vi "LVJSON Load.vi"(8 "error in (no error)":errorcluster, 11 "JSON in":string) -> (0 "error out":errorcluster, 1 "Empty?":bool, 3 "Root Element out":T1)   [LabVIEW 2018, in "labview_json.lvlib"]
uses:
  labview_json.lvlib
  Element Type.ctl
  Element.ctl
  <vilib>/regexp/Match Regular Expression.xnode
  <vilib>/ErrorRing/Error Ring.xnode
  <vilib>/Utility/error.llb/Error Cluster From Error Code.vi
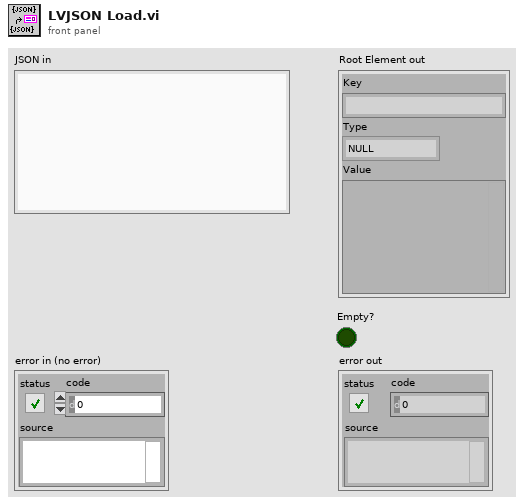
[diagram p1: front panel]
types:
  T1 = typedef "labview_json.lvlib/Element.ctl" = cluster{"Key":string, "Type":T2, "Value":variant}
  T2 = typedef "labview_json.lvlib/Element Type.ctl" = enum8{"NULL", "BOOL", "INT", "UINT", "FLOAT", "STRING", "ARRAY", "OBJECT", "SKIP"}
  T3 = cluster{"Kind":enum8{"Root", "Object", "Array"}, "Name":string, "Values":T1[]}[]
  T4 = cluster{"Kind":enum8{"Root", "Object", "Array"}, "Name":string, "Values":T1[]}
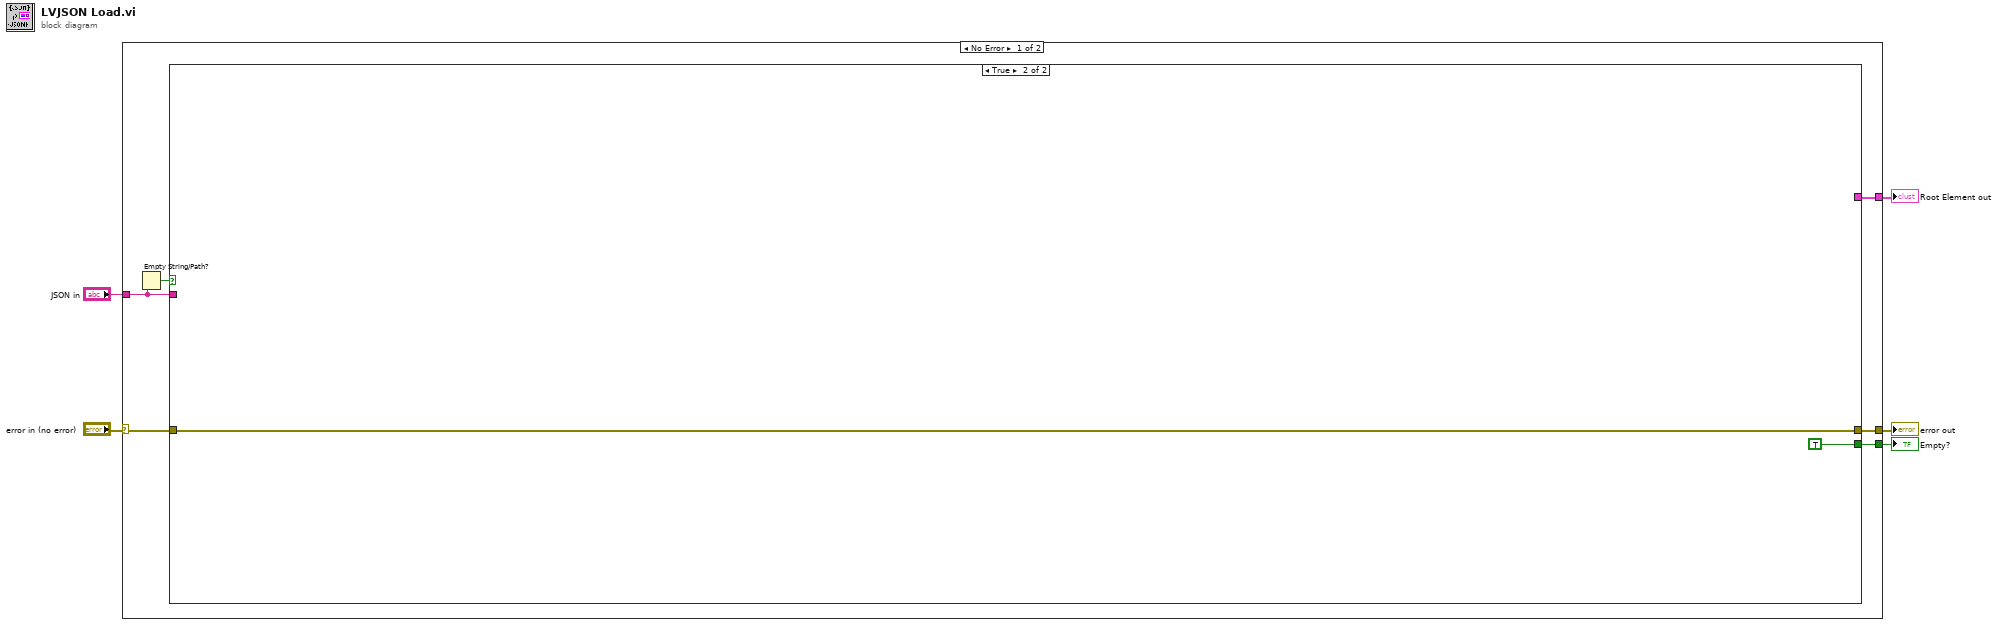
[diagram p0: block diagram]
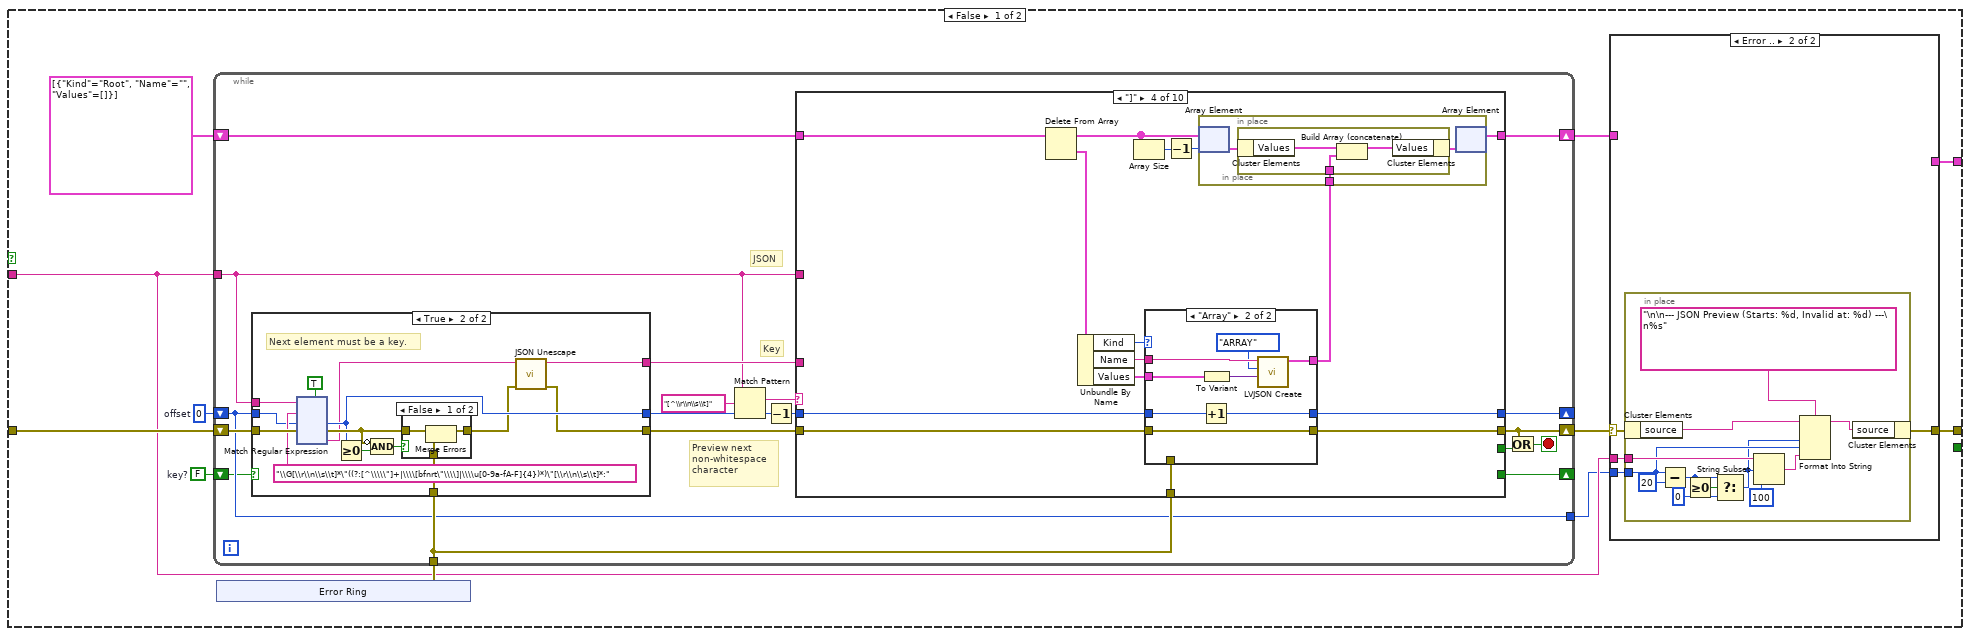
[diagram p2: hidden frame]
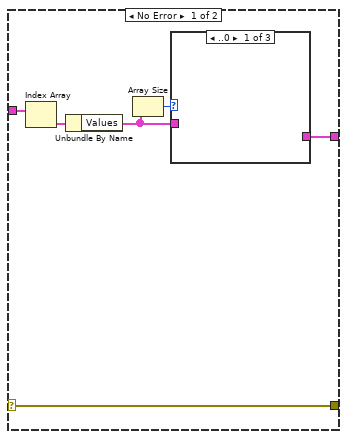
[diagram p3: hidden frame]
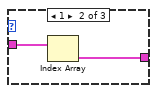
[diagram p4: hidden frame]
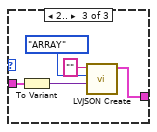
[diagram p5: hidden frame]
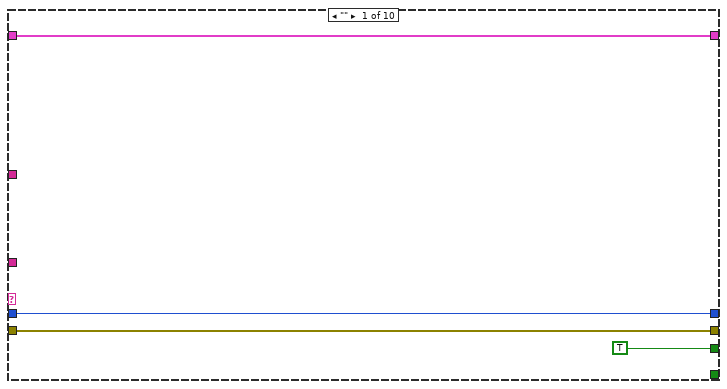
[diagram p8: hidden frame]
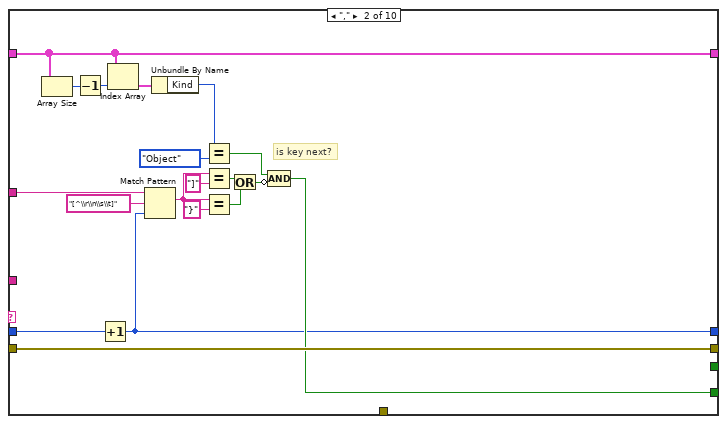
[diagram p9: hidden frame]
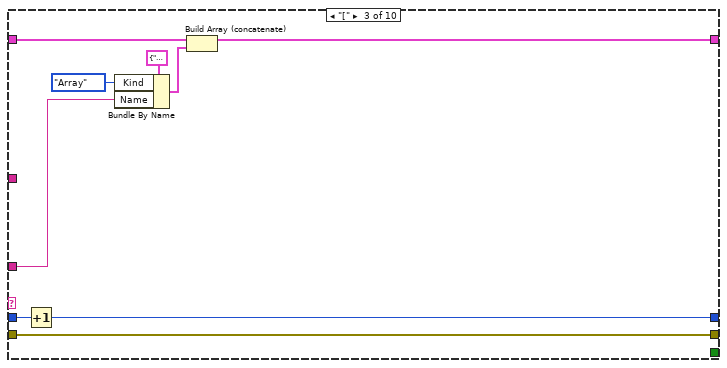
[diagram p10: hidden frame]
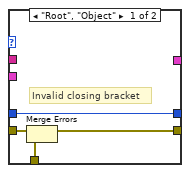
[diagram p11: hidden frame]
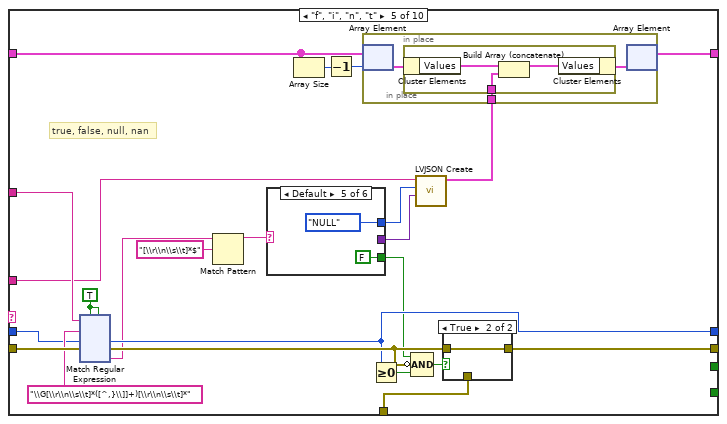
[diagram p12: hidden frame]
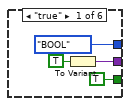
[diagram p13: hidden frame]
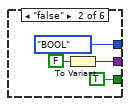
[diagram p14: hidden frame]
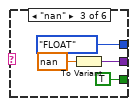
[diagram p15: hidden frame]
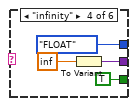
[diagram p16: hidden frame]
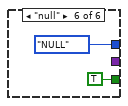
[diagram p17: hidden frame]
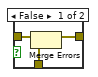
[diagram p18: hidden frame]
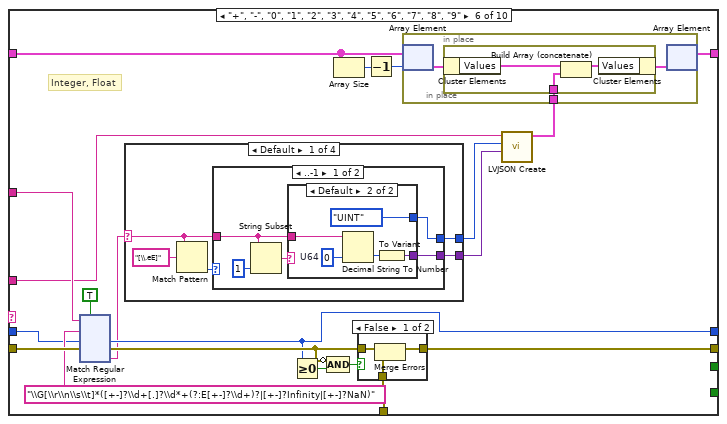
[diagram p19: hidden frame]
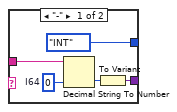
[diagram p20: hidden frame]
diagram:
  n1 = case shown="No Error" "error in (no error)" {
    selector: "error in (no error)" -> [w11 w839]
    tunnel: [w10 _] -> w4
    tunnel: [w9 w839] -> w3
    tunnel: "JSON in" -> [w8 _]
    tunnel: [w6 _] -> w1
    frame No Error {
      n2 = Empty String/Path?(string/path=w8) -> (empty?=w7:bool)
      n3 = case shown="True" w7 {
        tunnel: w11 -> [w21 w838]
        tunnel: [w12 _] -> w10
        tunnel: [w18 w838] -> w9
        tunnel: w8 -> [w16 _]
        tunnel: [_ TRUE] -> w6
        frame False {
          w22 = 0  # offset
          w14 = FALSE  # key?
          n4 = xnode "Error Ring"() -> ("error out"=w20:errorcluster)
          n5 = while {
            tunnel: w16 -> [w64]
            shift-right: [w74] -> w13
            shift-left: T3 [{"Kind"=enum."Root", "Name"="", "Values"=[]}] ("Context") -> [w73]
            shift-right: [w72] -> _
            shift-left: w22 -> [w58]
            shift-right: [w61] -> w17
            shift-left: w21 -> [w71]
            tunnel: w20 -> [w63]
            tunnel: [w58] -> w15
            shift-right: [w56] -> _
            shift-left: w14 -> [w57]
            stop <- w60 stop-if-true
            # "JSON"
            # "Key"
            # "Preview next\nnon-whitespace\ncharacter"
            n6 = case shown="True" w57 {
              tunnel: w64 -> [_ w89]
              tunnel: w71 -> [w76 w88]
              tunnel: w58 -> [w75 w86]
              tunnel: [w76 w77] -> w67
              tunnel: w63 -> [_ w83]
              tunnel: [w75 w81] -> w69
              tunnel: [_ w79] -> w66
              frame False {
                # "No key"
                # "Next element can be anything"
              }
              frame True {
                # "Next element must be a key."
                n7 = xnode "Match Regular Expression"("input string"=w89, "regular expression"="\\G[\\r\\n\\s\\t]*\"((?:[^\\\\\"]+|\\\\[bfnrt\"\\\\]|\\\\u[0-9a-fA-F]{4})*)\"[\\r\\n\\s\\t]*:", "offset (0)"=w86, "error in"=w88, "multiline? (F)"=TRUE) -> ("offset past match"=w81:i32, "error out"=w82:errorcluster, "submatch 1"=w80:string)  [unwired: 1 in, 3 out]
                n8 = Greater Or Equal To 0?(x=w81) -> (x >= 0?=w85:bool)
                n9 = Compound Arithmetic op=AND(invert w82, w85) -> (w84:bool)
                n10 = case shown="False" w84 {
                  tunnel: w83 -> [w91 _]
                  tunnel: w82 -> [w93 w94]
                  tunnel: [w92 w94] -> w78
                  frame False {
                    n11 = Merge Errors(w93, w91) -> (w92:errorcluster)
                  }
                  frame True {
                  }
                }
                n12 = call "JSON Unescape.vi"("error in (no error)"=w78, "Escaped String"=w80) -> ("error out"=w77:errorcluster, "String out"=w79:string)  [unwired: 7 in, 1 out]
              }
            }
            n13 = Match Pattern(string=w64, regular expression="[^\\r\\n\\s\\t]", offset (0)=w69) -> (match substring=w68:string, offset past match=w65:i32)  [unwired: 2 out]
            n14 = Decrement(x=w65) -> (x-1=w62:i32)
            n15 = case shown="\"]\"" w68 {
              tunnel: [TRUE _ _ _ _ _ _ _ _ _] -> w59
              tunnel: w64 -> [_ w222 _ _ w296 w465 w650 w790 _ _]
              tunnel: w62 -> [w215 w221 w240 w248 w287 w456 w643 w793 w801 w834]
              tunnel: [w216 w236 w244 w255 w299 w468 w653 w797 w808 w836] -> w74
              tunnel: w73 -> [w216 w236 w245 w260 w298 w467 w652 w798 w813 w836]
              tunnel: [w215 w218 w238 w249 w289 w458 w645 w786 w802 w834] -> w72
              tunnel: [w214 w220 w239 w252 w288 w457 w644 w792 w805 w833] -> w61
              tunnel: w67 -> [w214 w220 w239 w251 w297 w466 w651 w792 w804 w835]
              tunnel: w66 -> [_ _ w242 _ w282 w454 w638 w795 _ _]
              tunnel: w63 -> [_ _ _ w250 w290 w459 w646 _ w803 w832]
              tunnel: [_ w219 _ _ _ _ _ w787 _ _] -> w56
              frame "" {
              }
              frame "," {
                # "is key next?"
                n16 = Array Size(array=w236) -> (size(s)=w235:i32)
                n17 = Decrement(x=w235) -> (x-1=w234:i32)
                n18 = Increment(x=w221) -> (x+1=w218:i32)
                n19 = Index Array(array=w236, index=w234) -> (element=w233:T4)
                n20 = Match Pattern(string=w222, regular expression="[^\\r\\n\\s\\t]", offset (0)=w218) -> (match substring=w225:string)  [unwired: 3 out]
                n21 = Unbundle By Name(w233) -> ("Kind"=w224:enum8{"Root", "Object", "Array"})
                n22 = Equal?(x=w224, y=enum8{"Root", "Object", "Array"}."Object") -> (x = y?=w228:bool)
                n23 = Equal?(x=w225, y="]") -> (x = y?=w230:bool)
                n24 = Equal?(x=w225, y="}") -> (x = y?=w229:bool)
                n25 = Or(x=w230, y=w229) -> (x .or. y?=w227:bool)
                n26 = Compound Arithmetic op=AND(w228, invert w227) -> (w219:bool)
              }
              frame "[" {
                n27 = Increment(x=w240) -> (x+1=w238:i32)
                n28 = Bundle By Name(cluster=T4 {"Kind"=enum."Root", "Name"="", "Values"=[]} ("Context"), "Kind"=enum8{"Root", "Object", "Array"}."Array", "Name"=w242) -> (w243:T4)
                n29 = Build Array (concatenate)(w245, w243) -> (w244:T3)
              }
              frame "]" {
                n30 = Delete From Array(array=w260) -> (deleted portion=w259:T4, array with subset deleted=w256:T3)  [unwired: 2 in]
                n31 = Unbundle By Name(w259) -> ("Kind"=w254:enum8{"Root", "Object", "Array"}, "Name"=w247:string, "Values"=w253:T1[])
                n32 = Array Size(array=w256) -> (size(s)=w258:i32)
                n33 = case shown="\"Array\"" w254 {
                  tunnel: w253 -> [_ w269]
                  tunnel: [w263 w271] -> w252
                  tunnel: w251 -> [w264 w271]
                  tunnel: w250 -> [w262 _]
                  tunnel: [w261 w270] -> w249
                  tunnel: w248 -> [w261 w272]
                  tunnel: [_ w266] -> w246
                  tunnel: w247 -> [_ w267]
                  frame "Root", "Object" {
                    # "Invalid closing bracket"
                    n34 = Merge Errors(w264, w262) -> (w263:errorcluster)
                  }
                  frame "Array" {
                    n35 = Increment(x=w272) -> (x+1=w270:i32)
                    n36 = To Variant(anything=w269) -> (Variant=w268:variant)
                    n37 = call "LVJSON Create.vi"("Variant (Void=Default Type)"=w268, "Type"=Element_Type."ARRAY", "Key"=w267) -> ("Element out"=w266:T1)  [unwired: 8 in]
                  }
                }
                n38 = Decrement(x=w258) -> (x-1=w257:i32)
                n39 = in-place {
                  in-place-border: w246 -> [w274]
                  n40 = in-place-array #1(w256, w257) -> (w275:T4)
                  n41 = in-place {
                    in-place-border: w274 -> [w276]
                    n42 = in-place-cluster #2(w275) -> ("Values"=w278:T1[])
                    n43 = Build Array (concatenate)(w278, w276) -> (w277:T1[])
                    n44 = in-place-cluster #2("Values"=w277) -> (w273:T4)
                  }
                  n45 = in-place-array #1(w273) -> (w255:T3)  [unwired: 1 out]
                }
              }
              frame "f", "i", "n", "t" {
                w294 = TRUE ("ignore case? (F)")
                # "true, false, null, nan"
                n46 = xnode "Match Regular Expression"("input string"=w296, "regular expression"="\\G[\\r\\n\\s\\t]*([^,}\\]]+)[\\r\\n\\s\\t]*", "offset (0)"=w287, "error in"=w297, "ignore case? (F)"=w294, "multiline? (F)"=w294) -> ("offset past match"=w289:i32, "error out"=w291:errorcluster, "submatch 1"=w284:string)  [unwired: 3 out]
                n47 = Match Pattern(string=w284, regular expression="[\\r\\n\\s\\t]*$") -> (before substring=w283:string)  [unwired: 1 in, 3 out]
                n48 = case shown="Default" w283 {
                  tunnel: [Element_Type."BOOL" ("Type") Element_Type."BOOL" ("Type") Element_Type."FLOAT" ("Type") Element_Type."FLOAT" ("Type") Element_Type."NULL" ("Type") Element_Type."NULL" ("Type")] -> w281
                  tunnel: [w303 w307 w312 w316 _ _] -> w280
                  tunnel: [TRUE TRUE TRUE TRUE FALSE TRUE] -> w286
                  frame "true" {
                    n49 = To Variant(anything=TRUE) -> (Variant=w303:variant)
                  }
                  frame "false" {
                    n50 = To Variant(anything=FALSE) -> (Variant=w307:variant)
                  }
                  frame "nan" {
                    n51 = To Variant(anything=nan) -> (Variant=w312:variant)
                  }
                  frame "infinity" {
                    n52 = To Variant(anything=inf) -> (Variant=w316:variant)
                  }
                  frame Default {
                  }
                  frame "null" {
                  }
                }
                n53 = Array Size(array=w298) -> (size(s)=w301:i32)
                n54 = Decrement(x=w301) -> (x-1=w300:i32)
                n55 = Greater Or Equal To 0?(x=w289) -> (x >= 0?=w292:bool)
                n56 = Compound Arithmetic op=AND(w286, invert w291, w292) -> (w293:bool)
                n57 = call "LVJSON Create.vi"("Variant (Void=Default Type)"=w280, "Type"=w281, "Key"=w282) -> ("Element out"=w279:T1)  [unwired: 8 in]
                n58 = in-place {
                  in-place-border: w279 -> [w446]
                  n59 = in-place-array #3(w298, w300) -> (w447:T4)
                  n60 = in-place {
                    in-place-border: w446 -> [w448]
                    n61 = in-place-cluster #4(w447) -> ("Values"=w450:T1[])
                    n62 = Build Array (concatenate)(w450, w448) -> (w449:T1[])
                    n63 = in-place-cluster #4("Values"=w449) -> (w445:T4)
                  }
                  n64 = in-place-array #3(w445) -> (w299:T3)  [unwired: 1 out]
                }
                n65 = case shown="True" w293 {
                  tunnel: w290 -> [w322 _]
                  tunnel: w291 -> [w324 w325]
                  tunnel: [w323 w325] -> w288
                  frame False {
                    n66 = Merge Errors(w324, w322) -> (w323:errorcluster)
                  }
                  frame True {
                  }
                }
              }
              frame "+", "-", "0", "1", "2", "3", "4", "5", "6", "7", "8", "9" {
                # "Integer, Float"
                n67 = xnode "Match Regular Expression"("input string"=w465, "regular expression"="\\G[\\r\\n\\s\\t]*([+-]?\\d+[.]?\\d*+(?:E[+-]?\\d+)?|[+-]?Infinity|[+-]?NaN)", "offset (0)"=w456, "error in"=w466, "ignore case? (F)"=TRUE) -> ("offset past match"=w458:i32, "error out"=w460:errorcluster, "submatch 1"=w455:string)  [unwired: 1 in, 3 out]
                n68 = case shown="Default" w455 {
                  selector: w455 -> [w473 _ _ _]
                  tunnel: [w471 Element_Type."FLOAT" ("Type") Element_Type."FLOAT" ("Type") Element_Type."FLOAT" ("Type")] -> w453
                  tunnel: [w472 w497 w500 w503] -> w452
                  frame Default {
                    n69 = Match Pattern(string=w473, regular expression="[\\.eE]") -> (offset past match=w475:i32)  [unwired: 1 in, 3 out]
                    n70 = case shown="..-1" w475 {
                      tunnel: w473 -> [w479 w495]
                      tunnel: [w478 w492] -> w472
                      tunnel: [w476 Element_Type."FLOAT" ("Type")] -> w471
                      frame ..-1 {
                        n71 = String Subset(string=w479, length (rest)=1 ("length (rest)")) -> (substring=w477:string)  [unwired: 1 in]
                        n72 = case shown="Default" w477 {
                          tunnel: w479 -> [w485 w490]
                          tunnel: [w482 w487] -> w478
                          tunnel: [Element_Type."INT" ("Type") Element_Type."UINT" ("Type")] -> w476
                          frame "-" {
                            w484 = i64 0  # I64
                            n73 = Decimal String To Number(string=w485, default (0L)=w484) -> (number=w483:i64)  [unwired: 1 in, 1 out]
                            n74 = To Variant(anything=w483) -> (Variant=w482:variant)
                          }
                          frame Default {
                            w489 = u64 0  # U64
                            n75 = Decimal String To Number(string=w490, default (0L)=w489) -> (number=w488:u64)  [unwired: 1 in, 1 out]
                            n76 = To Variant(anything=w488) -> (Variant=w487:variant)
                          }
                        }
                      }
                      frame 0.. {
                        w494 = 0.0  # DBL
                        n77 = Fract/Exp String To Number(string=w495, default (0 dbl)=w494) -> (number=w493:dbl)  [unwired: 2 in, 1 out]
                        n78 = To Variant(anything=w493) -> (Variant=w492:variant)
                      }
                    }
                  }
                  frame "+Infinity", "Infinity" {
                    n79 = To Variant(anything=inf) -> (Variant=w497:variant)
                  }
                  frame "-Infinity" {
                    n80 = To Variant(anything=-inf) -> (Variant=w500:variant)
                  }
                  frame "+NaN", "-NaN", "NaN" {
                    n81 = To Variant(anything=nan) -> (Variant=w503:variant)
                  }
                }
                n82 = Greater Or Equal To 0?(x=w458) -> (x >= 0?=w461:bool)
                n83 = Compound Arithmetic op=AND(invert w460, w461) -> (w462:bool)
                n84 = Array Size(array=w467) -> (size(s)=w470:i32)
                n85 = case shown="False" w462 {
                  tunnel: w459 -> [w505 _]
                  tunnel: w460 -> [w507 w508]
                  tunnel: [w506 w508] -> w457
                  frame False {
                    n86 = Merge Errors(w507, w505) -> (w506:errorcluster)
                  }
                  frame True {
                  }
                }
                n87 = Decrement(x=w470) -> (x-1=w469:i32)
                n88 = call "LVJSON Create.vi"("Variant (Void=Default Type)"=w452, "Type"=w453, "Key"=w454) -> ("Element out"=w451:T1)  [unwired: 8 in]
                n89 = in-place {
                  in-place-border: w451 -> [w629]
                  n90 = in-place-array #5(w467, w469) -> (w630:T4)
                  n91 = in-place {
                    in-place-border: w629 -> [w631]
                    n92 = in-place-cluster #6(w630) -> ("Values"=w633:T1[])
                    n93 = Build Array (concatenate)(w633, w631) -> (w632:T1[])
                    n94 = in-place-cluster #6("Values"=w632) -> (w628:T4)
                  }
                  n95 = in-place-array #5(w628) -> (w468:T3)  [unwired: 1 out]
                }
              }
              frame "\"" {
                # "String"
                n96 = Array Size(array=w652) -> (size(s)=w655:i32)
                n97 = xnode "Match Regular Expression"("input string"=w650, "regular expression"="\\G[\\r\\n\\s\\t]*\"((?:[^\\\\\"]+|\\\\[bfnrt\"\\\\]|\\\\u[0-9a-fA-F]{4})*)\"", "offset (0)"=w643, "error in"=w651, "multiline? (F)"=TRUE ("ignore case? (F)")) -> ("offset past match"=w645:i32, "error out"=w640:errorcluster, "submatch 1"=w641:string)  [unwired: 1 in, 3 out]
                n98 = Decrement(x=w655) -> (x-1=w654:i32)
                n99 = call "JSON Unescape.vi"("error in (no error)"=w640, "Escaped String"=w641) -> ("error out"=w639:errorcluster, "String out"=w636:string)  [unwired: 7 in, 1 out]
                n100 = To Variant(anything=w636) -> (Variant=w634:variant)
                n101 = call "LVJSON Create.vi"("Variant (Void=Default Type)"=w634, "Type"=Element_Type."STRING", "Key"=w638) -> ("Element out"=w635:T1)  [unwired: 8 in]
                n102 = in-place {
                  in-place-border: w635 -> [w780]
                  n103 = in-place-array #7(w652, w654) -> (w781:T4)
                  n104 = in-place {
                    in-place-border: w780 -> [w782]
                    n105 = in-place-cluster #8(w781) -> ("Values"=w784:T1[])
                    n106 = Build Array (concatenate)(w784, w782) -> (w783:T1[])
                    n107 = in-place-cluster #8("Values"=w783) -> (w779:T4)
                  }
                  n108 = in-place-array #7(w779) -> (w653:T3)  [unwired: 1 out]
                }
                n109 = Greater Or Equal To 0?(x=w645) -> (x >= 0?=w647:bool)
                n110 = Compound Arithmetic op=AND(invert w639, w647) -> (w648:bool)
                n111 = case shown="False" w648 {
                  tunnel: w646 -> [w656 _]
                  tunnel: w639 -> [w658 w659]
                  tunnel: [w657 w659] -> w644
                  frame False {
                    n112 = Merge Errors(w658, w656) -> (w657:errorcluster)
                  }
                  frame True {
                  }
                }
              }
              frame "{" {
                # "Is key next?"
                n113 = Increment(x=w793) -> (x+1=w786:i32)
                n114 = Bundle By Name(cluster=T4 {"Kind"=enum."Root", "Name"="", "Values"=[]} ("Context"), "Kind"=enum8{"Root", "Object", "Array"}."Object", "Name"=w795) -> (w796:T4)
                n115 = Match Pattern(string=w790, regular expression="[^\\r\\n\\s\\t]", offset (0)=w786) -> (match substring=w789:string)  [unwired: 3 out]
                n116 = Build Array (concatenate)(w798, w796) -> (w797:T3)
                n117 = Not Equal?(x=w789, y="}") -> (x != y?=w787:bool)
              }
              frame "}" {
                n118 = Delete From Array(array=w813) -> (deleted portion=w812:T4, array with subset deleted=w809:T3)  [unwired: 2 in]
                n119 = Unbundle By Name(w812) -> ("Kind"=w807:enum8{"Root", "Object", "Array"}, "Name"=w800:string, "Values"=w806:T1[])
                n120 = Array Size(array=w809) -> (size(s)=w811:i32)
                n121 = case shown="\"Object\"" w807 {
                  tunnel: w806 -> [_ w822]
                  tunnel: [w816 w824] -> w805
                  tunnel: w804 -> [w817 w824]
                  tunnel: w803 -> [w815 _]
                  tunnel: [w814 w823] -> w802
                  tunnel: w801 -> [w814 w825]
                  tunnel: [_ w818] -> w799
                  tunnel: w800 -> [_ w820]
                  frame "Root", "Array" {
                    # "Invalid closing bracket"
                    n122 = Merge Errors(w817, w815) -> (w816:errorcluster)
                  }
                  frame "Object" {
                    n123 = Increment(x=w825) -> (x+1=w823:i32)
                    n124 = To Variant(anything=w822) -> (Variant=w821:variant)
                    n125 = call "LVJSON Create.vi"("Variant (Void=Default Type)"=w821, "Type"=Element_Type."OBJECT", "Key"=w820) -> ("Element out"=w818:T1)  [unwired: 8 in]
                  }
                }
                n126 = Decrement(x=w811) -> (x-1=w810:i32)
                n127 = in-place {
                  in-place-border: w799 -> [w827]
                  n128 = in-place-array #9(w809, w810) -> (w828:T4)
                  n129 = in-place {
                    in-place-border: w827 -> [w829]
                    n130 = in-place-cluster #10(w828) -> ("Values"=w831:T1[])
                    n131 = Build Array (concatenate)(w831, w829) -> (w830:T1[])
                    n132 = in-place-cluster #10("Values"=w830) -> (w826:T4)
                  }
                  n133 = in-place-array #9(w826) -> (w808:T3)  [unwired: 1 out]
                }
              }
              frame Default {
                # "Invalid value"
                n134 = Merge Errors(w835, w832) -> (w833:errorcluster)
              }
            }
            n135 = Or(x=w61, y=w59) -> (x .or. y?=w60:bool)
          }
          n136 = case shown="Error .." w17 {
            selector: w17 -> [w28 w39]
            tunnel: [w28 w36] -> w18
            tunnel: w16 -> [_ w38]
            tunnel: w15 -> [_ w37]
            tunnel: w13 -> [w24 _]
            tunnel: [w23 _] -> w12
            frame No Error {
              n137 = Index Array(array=w24) -> (element=w26:T4)  [unwired: 1 in]
              n138 = Unbundle By Name(w26) -> ("Values"=w25:T1[])
              n139 = Array Size(array=w25) -> (size(s)=w27:i32)
              n140 = case shown="..0" w27 {
                tunnel: w25 -> [_ w30 w35]
                tunnel: [_ w29 w31] -> w23
                frame ..0 {
                }
                frame 1 {
                  n141 = Index Array(array=w30) -> (element=w29:T1)  [unwired: 1 in]
                }
                frame 2.. {
                  n142 = To Variant(anything=w35) -> (Variant=w34:variant)
                  n143 = call "LVJSON Create.vi"("Variant (Void=Default Type)"=w34, "Type"=Element_Type."ARRAY", "Key"="") -> ("Element out"=w31:T1)  [unwired: 8 in]
                }
              }
            }
            frame Error {
              n144 = in-place {
                in-place-border: w38 -> [w51]
                in-place-border: w37 -> [w41]
                n145 = in-place-cluster #11(w39) -> ("source"=w48:string)
                n146 = Subtract(x=w41, y=20 ("x")) -> (x-y=w44:i32)
                n147 = Greater Or Equal To 0?(x=w44) -> (x >= 0?=w45:bool)
                n148 = Select(t=w44, s=w45, f=0) -> (s? t:f=w40:i32)
                n149 = String Subset(string=w51, offset (0)=w40, length (rest)=100 ("length (rest)")) -> (substring=w42:string)
                n150 = Format Into String(format string="\n\n--- JSON Preview (Starts: %d, Invalid at: %d) ---\n%s", initial string=w48, w40, w41, w42) -> (resulting string=w47:string)  [unwired: 1 in, 1 out]
                n151 = in-place-cluster #11("source"=w47) -> (w36:errorcluster)
              }
            }
          }
        }
        frame True {
        }
      }
    }
    frame Error {
    }
  }
  "Root Element out" <- w4
  "error out" <- w3
  "Empty?" <- w1
